vi "getPosition.vi"() -> (2 "Latitude":dbl, 3 "Longitude":dbl)   [LabVIEW 2019]
uses:
  System.Device
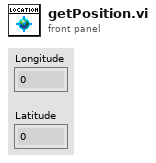
[diagram p1: front panel]
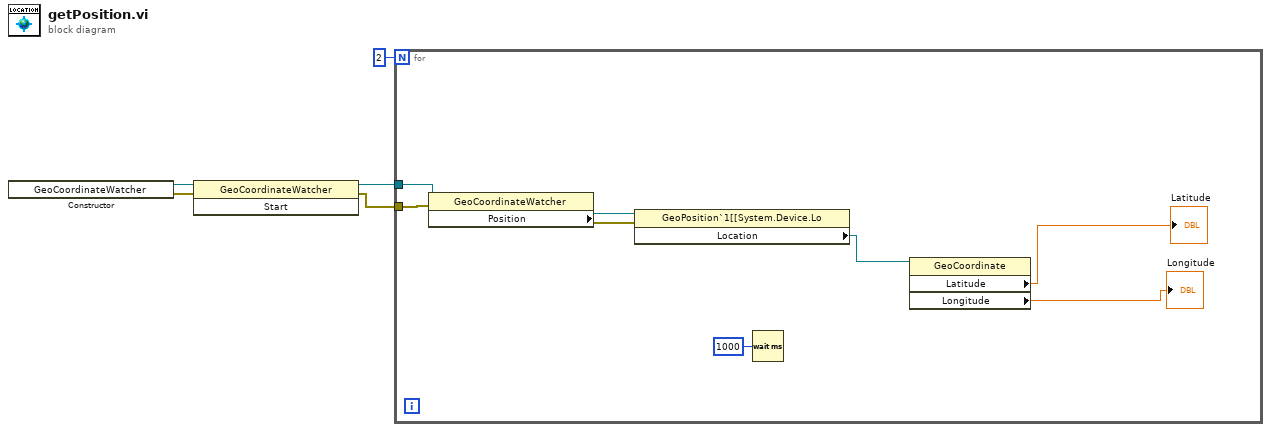
[diagram p0: block diagram]
diagram:
  n1 = constructor class="GeoCoordinateWatcher"() -> (reference out=w3:refnum<k24>, error out=w4:errorcluster)  [unwired: 3 in, 1 out]
  n2 = invoke class="GeoCoordinateWatcher" method="Start"(reference=w3, error in=w4) -> (reference out=w5:refnum<k24>, error out=w2:errorcluster)  [unwired: 1 in, 1 out]
  n3 = for {
    N: 2 -> [_]
    tunnel: w5 -> [w13]
    tunnel: w2 -> [w11]
    n4 = property class="GeoCoordinateWatcher"(reference=w13, error in=w11) -> (error out=w12:errorcluster, "Position"=w10:refnum<k24>)  [unwired: 1 out]
    n5 = property class="GeoPosition`1[[System.Device.Lo"(reference=w10, error in=w12) -> ("Location"=w9:refnum<k24>)  [unwired: 2 out]
    n6 = Wait (ms)(milliseconds to wait=u32 1000) -> ()  [unwired: 1 out]
    n7 = property class="GeoCoordinate"(reference=w9) -> ("Latitude"=→"Latitude":dbl, "Longitude"=→"Longitude":dbl)  [unwired: 1 in, 2 out]
  }
